vi "Request.vi"(8 "error in (no error)":errorcluster, 10 "Input":T1, 11 "Vision Receiver in":refnum<class "Vision Receiver.lvclass">) -> (0 "error out":errorcluster, 3 "Vision Receiver out":refnum<class "Vision Receiver.lvclass">)   [LabVIEW 2022 SP3]
uses:
  Vision Receiver.lvclass
  UDP Input.ctl
  Vision Receiver.lvclass/Vision Receiver.ctl
  UDP Reader/UDP Reader Messages/Request Msg/Request Msg.lvclass/Request Msg.ctl
  <vilib>/ActorFramework/Message Enqueuer/Message Enqueuer.lvclass/Message Enqueuer.ctl
  <vilib>/ActorFramework/Message Enqueuer/Enqueue.vi
  UDP Reader/UDP Reader Messages/Request Msg/Request Msg.lvclass
  C:/Program Files (x86)/National Instruments/LabVIEW 2022/vi.lib/ActorFramework/Message/Message.lvclass
  <vilib>/ActorFramework/Message Priority Queue/Priority Enqueue.vi
  C:/Program Files (x86)/National Instruments/LabVIEW 2022/vi.lib/MGI/Monitored Actor/Monitored Actor/Monitored Actor/Monitored Actor.lvclass
  C:/Program Files (x86)/National Instruments/LabVIEW 2022/vi.lib/ActorFramework/Actor/Actor.lvclass
  C:/Users/ebert/Documents/codes/ssl/repo/Phoenix Reborn/Vision Receiver/Vision Receiver/Vision Receiver.lvclass
  C:/Users/ebert/Documents/codes/ssl/repo/Phoenix Reborn/UDP Data Receiver/UDP Data Receiver/UDP Data Receiver.lvclass
  <vilib>/ActorFramework/Message Enqueuer/Message Enqueuer.lvclass
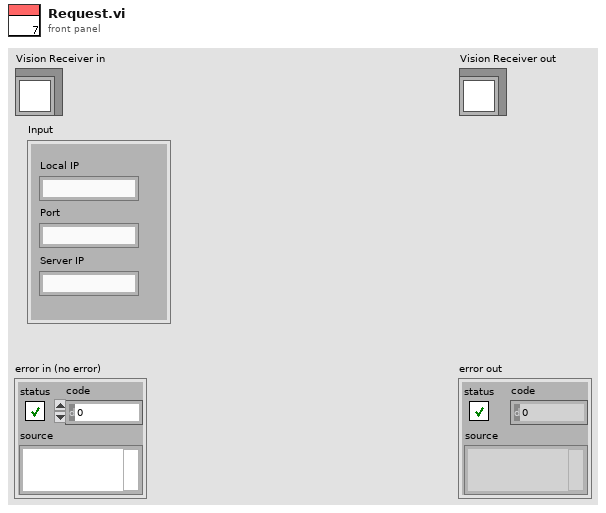
[diagram p1: front panel]
types:
  T1 = typedef "UDP Input.ctl" = cluster{"Local IP":string, "Port":string, "Server IP":string}
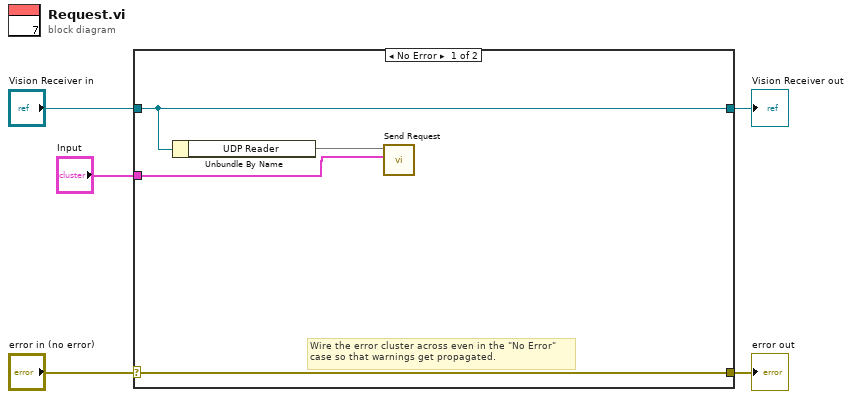
[diagram p0: block diagram]
diagram:
  n1 = case shown="No Error" "error in (no error)" {
    selector: "error in (no error)" -> [w9 w11]
    tunnel: [w9 w11] -> w4
    tunnel: [w8 w10] -> w2
    tunnel: "Vision Receiver in" -> [w8 w10]
    tunnel: "Input" -> [w6 _]
    frame No Error {
      # "Wire the error cluster across even in the \"No Error\"\ncase so that warnings get propagated."
      n2 = Unbundle By Name(w8) -> ("UDP Reader"=w7)
      n3 = call "Send Request.vi"("Input"=w6, "Message Enqueuer in"=w7) -> ()  [unwired: 8 in, 2 out]
    }
    frame Error {
    }
  }
  "error out" <- w4
  "Vision Receiver out" <- w2
